vi "UDP Test.vi"() -> ()   [LabVIEW 2018]
panel:
  out "unsigned byte array":u8[][](array[numeric])
  in  "connection ID out":refnum<k16>
  out "*(type *) &x":u8[](array[numeric])
  out "error out":errorcluster
  in  "stop":bool
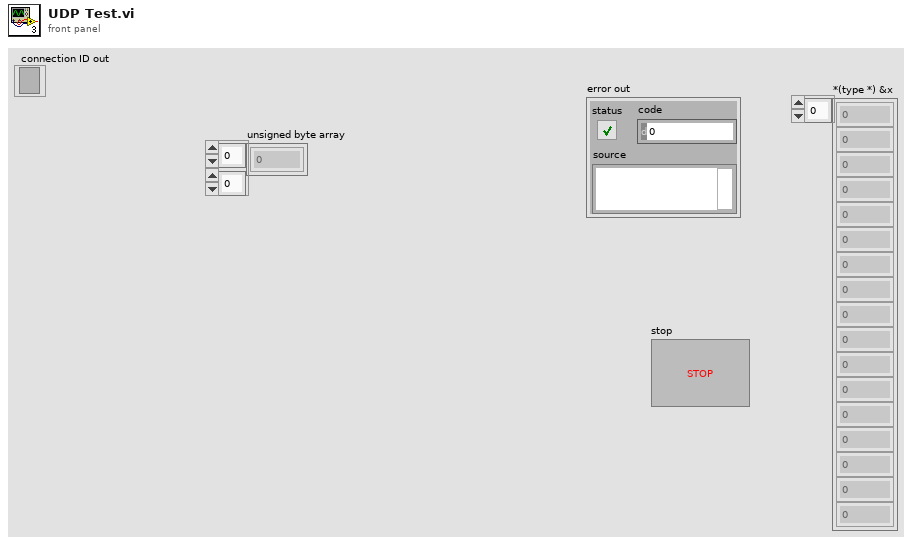
[diagram p1: front panel]
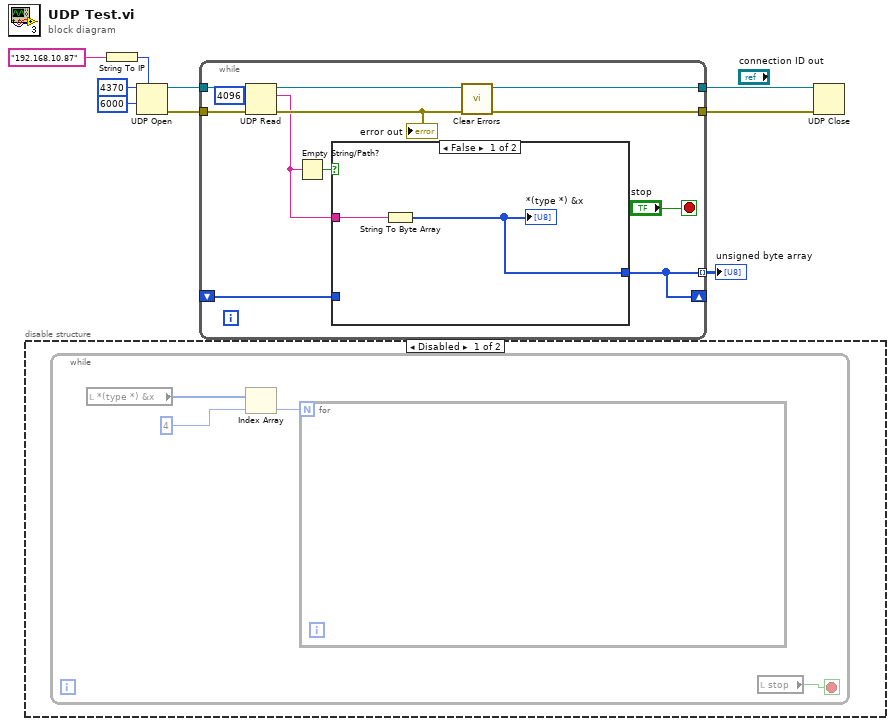
[diagram p0: block diagram]
diagram:
  n1 = disable-structure shown="Disabled" {
    frame Disabled {
      n2 = while {
        stop <- w13 stop-if-true
        n3 = local read "*(type *) &x"() -> (w11:u8[])
        n4 = Index Array(array=w11, index=4) -> (element=w10:u8)
        n5 = for {
          N: w10 -> [_]
        }
        n6 = local read "stop"() -> (w13:bool)
      }
    }
    frame Enabled {
    }
  }
  n7 = String To IP(1:"192.168.10.87") -> (0:w8:u32)
  n8 = UDP Open(7:w8, 9:6000 ("timeout ms (25000)"), 11:u16 4370 ("port")) -> (port=w5:refnum<k16>, 0:w4:errorcluster)  [unwired: 2 in, 1 out]
  n9 = while {
    tunnel: w5 -> [w24]
    tunnel: w4 -> [w23]
    tunnel: [w21] -> w3
    tunnel: [w20] -> w2
    tunnel: [w15] -> w1 mode=indexing
    shift-right: [w15] -> _
    shift-left: _ -> [w14]
    stop <- "stop" stop-if-true
    n10 = UDP Read(connection ID=w24, max size (548)=4096, 8:w23) -> (data out=w17:string, error out=w22:errorcluster, 3:w21:refnum<k16>)  [unwired: 1 in, 2 out]
    "error out" <- w22
    n11 = Empty String/Path?(string/path=w17) -> (empty?=w18:bool)
    n12 = case shown="False" w18 {
      tunnel: w17 -> [w26 _]
      tunnel: [w25 w27] -> w15
      tunnel: w14 -> [_ w27]
      frame False {
        n13 = String To Byte Array(string=w26) -> (unsigned byte array=w25:u8[])
        "*(type *) &x" <- w25
      }
      frame True {
      }
    }
    n14 = call <vilib>:"Clear Errors.vi"("error in (no error)"=w22) -> ("error out"=w20:errorcluster)  [unwired: 5 in, 1 out]
  }
  "unsigned byte array" <- w1
  n15 = UDP Close(connection ID=w3, 8:w2) -> ()  [unwired: 2 out]
